vi "Update Progress Bar.vi"(8 "error in":errorcluster, 11 "Peer Review":refnum<class "Peer Review.lvclass">) -> (0 "error out":errorcluster)   [LabVIEW 2020, in "Peer Review.lvclass"]
uses:
  Peer Review.lvclass
  Peer Review.lvclass/Peer Review.ctl
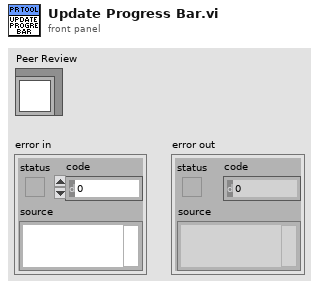
[diagram p1: front panel]
types:
  T1 = typedef "Peer Review.lvclass/File Info.ctl" = cluster{"File ID":i32, "Commit ID":i32, "Reviewed Hash":string, "Relative Path":string, "File Path":path, "File Checksum":string, "State":T2, "FP Changes":i32, "BD Changes":i32, "FP Bounds Error":dbl, "BD Bounds Error":dbl, "Lines Added":i32, "Lines Removed":i32, "Analysis Passes":i32, "Analysis Fails":i32, "Attribute Changes":i32, "Reentrancy State":string, "Cyclomatic Complexity":i32, "Node Count":i32, "Revision Number":u32, "LabVIEW Version":string, "Description":string, "Master Path":path, "Master Checksum":string, "VI Type":T3, "LabVIEW File":bool, "Review Complete":bool, "File Ref":refnum<vi>, "Master Revision":u32}
  T2 = typedef "Peer Review.lvclass/File State.ctl" = enum16{"Interrogation Needed", "Modified", "Deleted", "Added", "Matches Previous", "No Changes", "Moved", "Empty File"}
  T3 = typedef "Peer Review.lvclass/VI Type.ctl" = enum32{"invalid VI type", "Standard VI", "Control VI", "Global VI", "Polymorphic VI", "Configuration VI", "SubSystem", "Facade VI", "Method VI", "Statechart Diagram VI"}
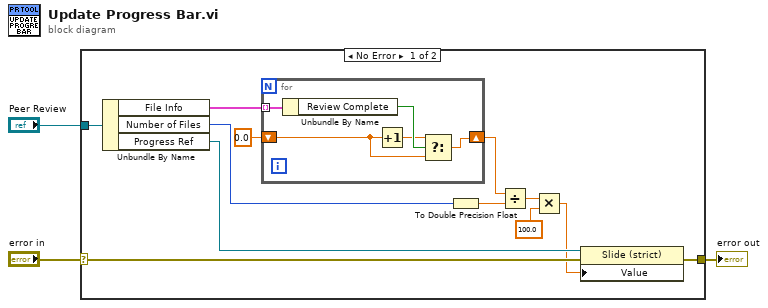
[diagram p0: block diagram]
diagram:
  n1 = case shown="No Error" "error in" {
    selector: "error in" -> [w10 w21]
    tunnel: [w9 w21] -> w2
    tunnel: "Peer Review" -> [w15 _]
    frame No Error {
      n2 = Unbundle By Name(w15) -> ("File Info"=w8:T1[], "Number of Files"=w4:i32, "Progress Ref"=w7:refnum<vi>)
      n3 = for {
        tunnel: w8 -> [w20] mode=indexing
        shift-right: [w16] -> w6
        shift-left: 0.0 -> [w17]
        n4 = Unbundle By Name(w20) -> ("Review Complete"=w19:bool)
        n5 = Increment(x=w17) -> (x+1=w18:dbl)
        n6 = Select(t=w18, s=w19, f=w17) -> (s? t:f=w16:dbl)
      }
      n7 = To Double Precision Float(number=w4) -> (double precision float=w13:dbl)
      n8 = Divide(x=w6, y=w13) -> (x/y=w12:dbl)
      n9 = Multiply(x=w12, y=100.0) -> (x*y=w5:dbl)
      n10 = property on="Property Node" class="Slide (strict)"(reference=w7, error in=w10, "Value"=w5) -> (error out=w9:errorcluster)  [unwired: 1 out]
    }
    frame Error {
    }
  }
  "error out" <- w2
